vi "Process.vi"(11 "obj":refnum<class "SimPump.lvclass">) -> ()   [LabVIEW 2019, in "SimPump.lvclass"]
doc: "Active object process.\n\nwww.sciware.com.au"
uses:
  SimPump.lvclass
  SimPump.lvclass/SimPump.ctl
panel:
  # "BSD License (http://www.opensource.org/licenses/bsd-license.php)"
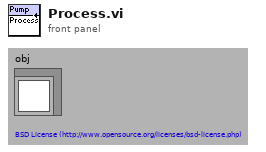
[diagram p1: front panel]
types:
  T1 = typedef "SimPump.lvclass/DataRef.ctl" = refnum<data-value>
  T2 = typedef "SimPump.lvclass/CmdQueueRef.ctl" = refnum<queue>
  T3 = typedef "SimPump.lvclass/CmdQueueType.ctl" = string
  T4 = typedef "SimPump.lvclass/DataMembers.ctl" = cluster{"flow rate":dbl, "volume to pump":dbl, "state":bool, "ti":u32, "t0":u32}
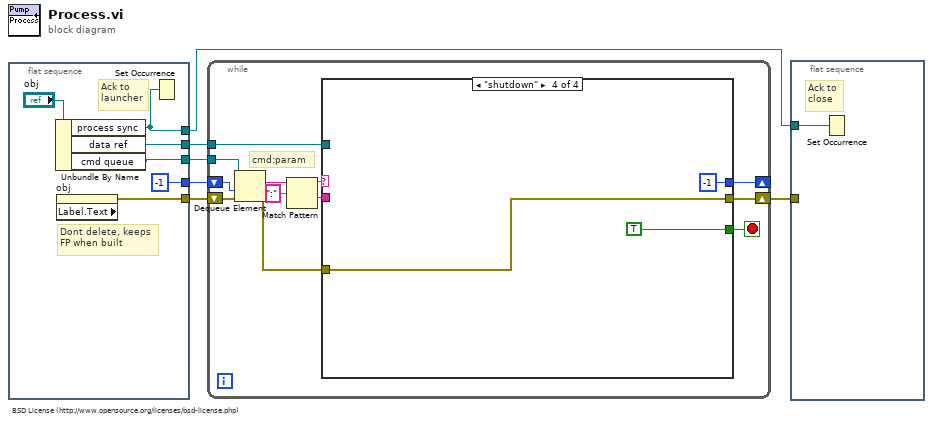
[diagram p0: block diagram]
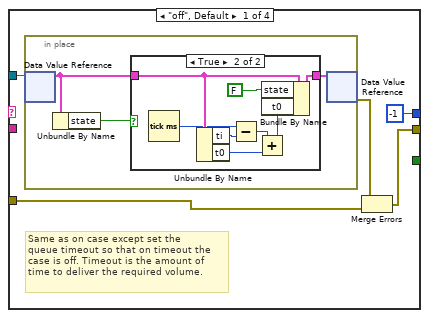
[diagram p2: hidden frame]
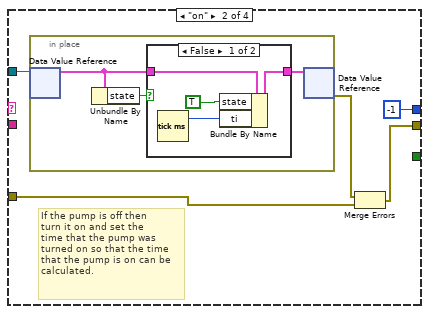
[diagram p4: hidden frame]
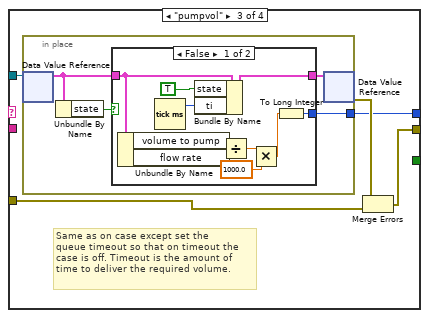
[diagram p6: hidden frame]
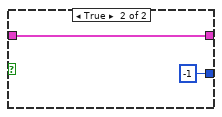
[diagram p7: hidden frame]
diagram:
  # "BSD License (http://www.opensource.org/licenses/bsd-license.php)"
  n1 = flat-sequence {
    tunnel: [w12] -> w6
    tunnel: [w11] -> w4
    tunnel: [w7] -> w3
    tunnel: [w10] -> w2
    tunnel: [-1 ("number")] -> w1
    frame #0 {
      # "Ack to\nlauncher"
      # "Dont delete, keeps\nFP when built"
      n2 = Unbundle By Name("obj") -> ("process sync"=w10:refnum<k4>, "data ref"=w11:T1, "cmd queue"=w12:T2)
      n3 = property on="obj" class="LVClassControl (strict)" props=["Label", "Text"]() -> (error out=w7:errorcluster)  [unwired: 2 in, 2 out]
      n4 = Set Occurrence(w10) -> ()
    }
  }
  n5 = while {
    tunnel: w6 -> [w24]
    shift-right: [w21] -> w5
    shift-left: w3 -> [w23]
    tunnel: w4 -> [w19]
    shift-right: [w13] -> _
    shift-left: w1 -> [w14]
    stop <- w20 stop-if-true
    # "cmd:param"
    n6 = Dequeue Element(queue=w24, timeout in ms (-1)=w14, error in (no error)=w23) -> (element=w18:T3, error out=w22:errorcluster)  [unwired: 2 out]
    n7 = Match Pattern(string=w18, regular expression=":") -> (before substring=w17:T3, after substring=w15:T3)  [unwired: 1 in, 2 out]
    n8 = case shown="\"shutdown\"" w17 {
      tunnel: [w26 w43 w56 w78] -> w21
      tunnel: w22 -> [w27 w44 w57 w78]
      tunnel: [_ _ _ TRUE] -> w20
      tunnel: w19 -> [w29 w46 w58 _]
      tunnel: w15 -> [_ _ _ _]
      tunnel: [-1 ("number") -1 ("number") w55 -1 ("number")] -> w13
      frame "off", Default {
        # "Same as on case except set the\nqueue timeout so that on timeout the\ncase is off. Timeout is the amount of\ntime to deliver the required volume."
        n9 = in-place {
          n10 = in-place-dvr #1(w29) -> (w31:T4)  [unwired: 1 out]
          n11 = Unbundle By Name(w31) -> ("state"=w30:bool)
          n12 = case shown="True" w30 {
            tunnel: [w33 w41] -> w32
            tunnel: w31 -> [w33 w39]
            frame False {
            }
            frame True {
              n13 = Tick Count (ms)() -> (millisecond timer value=w37:u32)
              n14 = Unbundle By Name(w39) -> ("ti"=w38:u32, "t0"=w35:u32)
              n15 = Subtract(x=w37, y=w38) -> (x-y=w36:u32)
              n16 = Add(x=w36, y=w35) -> (x+y=w34:u32)
              n17 = Bundle By Name(cluster=w39, "state"=FALSE, "t0"=w34) -> (w41:T4)
            }
          }
          n18 = in-place-dvr #1(w32) -> (w28:errorcluster)  [unwired: 1 out]
        }
        n19 = Merge Errors(w28, w27) -> (w26:errorcluster)
      }
      frame "on" {
        # "If the pump is off then\nturn it on and set the \ntime that the pump was\nturned on so that the time\nthat the pump is on can be\ncalculated."
        n20 = in-place {
          n21 = in-place-dvr #2(w46) -> (w48:T4)  [unwired: 1 out]
          n22 = Unbundle By Name(w48) -> ("state"=w47:bool)
          n23 = case shown="False" w47 {
            tunnel: [w53 w54] -> w49
            tunnel: w48 -> [w50 w54]
            frame False {
              n24 = Tick Count (ms)() -> (millisecond timer value=w51:u32)
              n25 = Bundle By Name(cluster=w50, "state"=TRUE, "ti"=w51) -> (w53:T4)
            }
            frame True {
            }
          }
          n26 = in-place-dvr #2(w49) -> (w45:errorcluster)  [unwired: 1 out]
        }
        n27 = Merge Errors(w45, w44) -> (w43:errorcluster)
      }
      frame "pumpvol" {
        # "Same as on case except set the\nqueue timeout so that on timeout the\ncase is off. Timeout is the amount of\ntime to deliver the required volume."
        n28 = in-place {
          in-place-border: [w62] -> w55
          n29 = in-place-dvr #3(w58) -> (w61:T4)  [unwired: 1 out]
          n30 = Unbundle By Name(w61) -> ("state"=w60:bool)
          n31 = case shown="False" w60 {
            tunnel: [w73 w75] -> w63
            tunnel: [w65 -1] -> w62
            tunnel: w61 -> [w64 w75]
            frame False {
              n32 = Unbundle By Name(w64) -> ("volume to pump"=w70:dbl, "flow rate"=w69:dbl)
              n33 = Tick Count (ms)() -> (millisecond timer value=w71:u32)
              n34 = Bundle By Name(cluster=w64, "state"=TRUE, "ti"=w71) -> (w73:T4)
              n35 = Divide(x=w70, y=w69) -> (x/y=w68:dbl)
              n36 = Multiply(x=w68, y=1000.0) -> (x*y=w66:dbl)
              n37 = To Long Integer(number=w66) -> (32bit integer=w65:i32)
            }
            frame True {
            }
          }
          n38 = in-place-dvr #3(w63) -> (w59:errorcluster)  [unwired: 1 out]
        }
        n39 = Merge Errors(w59, w57) -> (w56:errorcluster)
      }
      frame "shutdown" {
      }
    }
  }
  n40 = flat-sequence {
    tunnel: w5 -> [_]
    tunnel: w2 -> [w79]
    frame #0 {
      # "Ack to\nclose"
      n41 = Set Occurrence(w79) -> ()
    }
  }
